vi "TIFF camera test.vi"(8 "Gain":i32 min=0 max=2000 step=1, 9 "Exposure time (ms)":dbl=100.0 min=1.0 max=10000.0 step=1.0) -> (2 "Image out":T1(plugin-control))   [LabVIEW 2017]
uses:
  <vilib>/vision/Image Controls.llb/IMAQ Image.ctl
panel:
  in  "TIF file path":path=path "c:/test.avi"
  in  "stop":bool
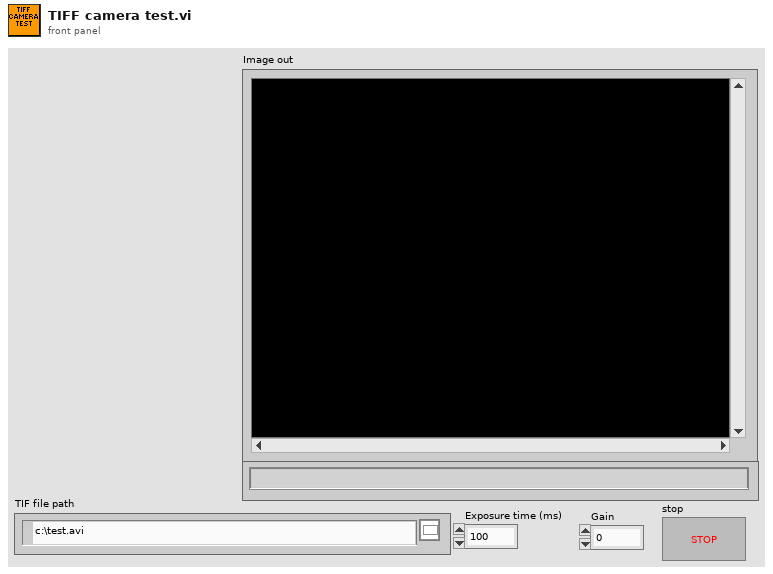
[diagram p1: front panel]
types:
  T1 = typedef "IMAQ Image.ctl" = refnum<image>
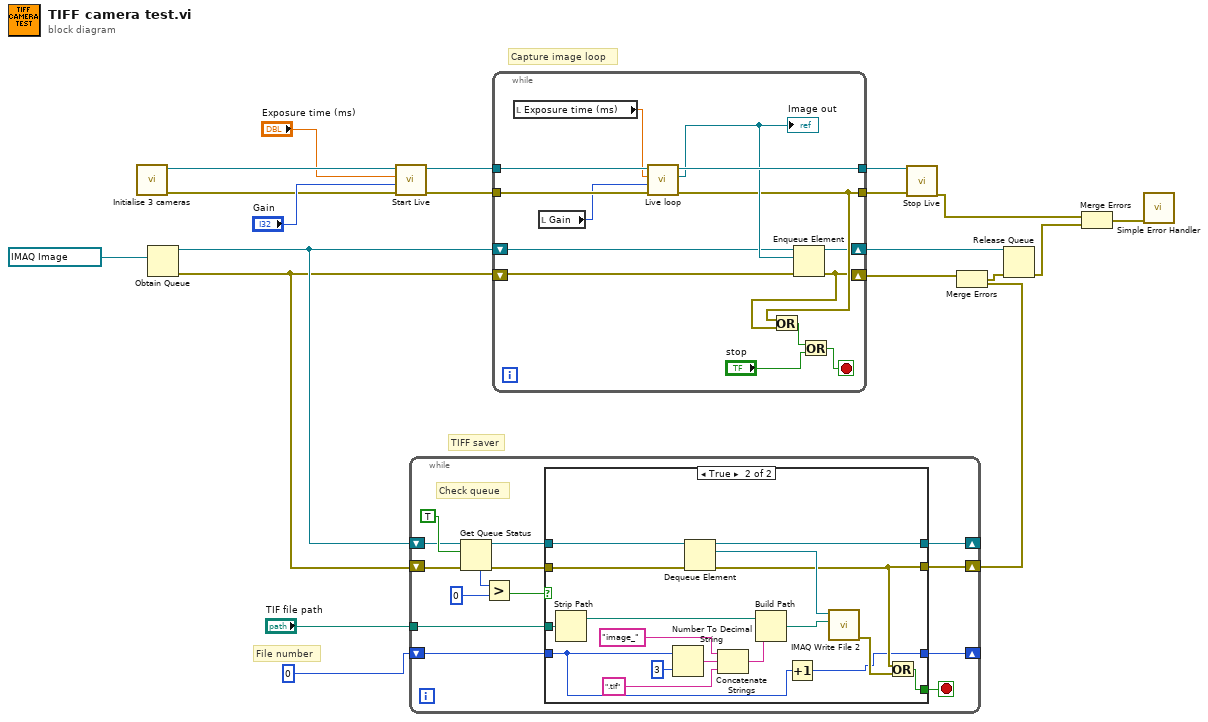
[diagram p0: block diagram]
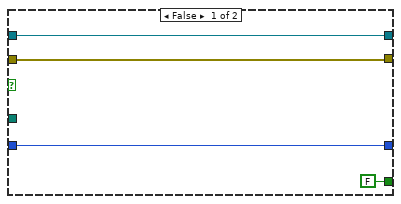
[diagram p2: hidden frame]
diagram:
  # "File number"
  # "TIFF saver"
  # "Capture image loop"
  n1 = call "Initialise 3 cameras.vi"() -> ("Error Out"=w17:errorcluster, "Red camera ref"=w20:refnum<k24>)  [unwired: 8 in, 2 out]
  n2 = Obtain Queue(element data type=T1 refnum ("Image out")) -> (queue out=w5:refnum<queue>, error out=w4:errorcluster)  [unwired: 4 in, 1 out]
  n3 = call "Start Live.vi"("Error In"=w17, "Gain in"="Gain", "Exposure time (ms)"="Exposure time (ms)", "Camera reference in"=w20) -> ("Error Out"=w13:errorcluster, "Camera reference out"=w14:refnum<k24>)  [unwired: 5 in]
  n4 = while {
    shift-right: [w34] -> _
    shift-left: w5 -> [w21]
    shift-right: [w31] -> w3
    shift-left: w4 -> [w24]
    tunnel: "TIF file path" -> [w33]
    shift-right: [w26] -> _
    shift-left: 0 -> [w30]
    stop <- w32 stop-if-true
    # "Check queue"
    n5 = Get Queue Status(queue=w21, return elements? (F)=TRUE, error in (no error)=w24) -> (queue out=w22:refnum<queue>, error out=w23:errorcluster, # elements in queue=w28:i32)  [unwired: 5 out]
    n6 = Greater?(x=w28, y=0) -> (0:w25:bool)
    n7 = case shown="True" w25 {
      tunnel: w22 -> [w38 w55]
      tunnel: w23 -> [w37 w54]
      tunnel: [w38 w53] -> w34
      tunnel: w33 -> [_ w52]
      tunnel: [FALSE w43] -> w32
      tunnel: [w37 w42] -> w31
      tunnel: w30 -> [w36 w40]
      tunnel: [w36 w39] -> w26
      frame False {
      }
      frame True {
        n8 = Strip Path(path=w52) -> (stripped path=w51:path)  [unwired: 1 out]
        n9 = Number To Decimal String(number=w40, width (-)=i16 3) -> (decimal integer string=w49:string)
        n10 = Dequeue Element(queue=w55, error in (no error)=w54) -> (queue out=w53:refnum<queue>, element=w44:T1, error out=w42:errorcluster)  [unwired: 1 in, 1 out]
        n11 = Concatenate Strings("image_", w49, ".tif") -> (w46:string)
        n12 = Build Path(base path=w51, name or relative path=w46) -> (appended path=w45:path)
        n13 = Increment(x=w40) -> (x+1=w39:i32)
        n14 = call-poly "IMAQ Write File 2"("File Path"=w45, "Image"=w44) -> ("error out"=w41:errorcluster)  [unwired: 8 in, 1 out]
        n15 = Or(x=w42, y=w41) -> (x .or. y?=w43:bool)
      }
    }
  }
  n16 = while {
    tunnel: [w58] -> w16
    tunnel: [w69] -> w15
    tunnel: w14 -> [w68]
    tunnel: w13 -> [w67]
    shift-right: [w57] -> w11
    shift-left: w5 -> [w60]
    shift-right: [w56] -> w9
    shift-left: w4 -> [w59]
    stop <- w62 stop-if-true
    n17 = local read "Exposure time (ms)"() -> (w66:dbl)
    n18 = local read "Gain"() -> (w65:i32)
    n19 = call "Live loop.vi"("Error In"=w67, "Gain"=w65, "Exposure time (ms)"=w66, "Camera reference in"=w68) -> ("Error Out"=w58:errorcluster, "Image out"=w61:T1, "Camera reference out"=w69:refnum<k24>)  [unwired: 4 in]
    "Image out" <- w61
    n20 = Enqueue Element(queue=w60, element=w61, error in (no error)=w59) -> (queue out=w57:refnum<queue>, error out=w56:errorcluster)  [unwired: 1 in, 1 out]
    n21 = Or(x=w58, y=w56) -> (x .or. y?=w64:bool)
    n22 = Or(x=w64, y="stop") -> (x .or. y?=w62:bool)
  }
  n23 = call "Stop Live.vi"("Camera reference in"=w15, "Error In"=w16) -> ("Error Out"=w8:errorcluster)  [unwired: 16 in, 1 out]
  n24 = Merge Errors(w9, w3) -> (w10:errorcluster)
  n25 = Release Queue(queue=w11, error in (no error)=w10) -> (error out=w7:errorcluster)  [unwired: 1 in, 2 out]
  n26 = Merge Errors(w8, w7) -> (w6:errorcluster)
  n27 = call <vilib>:"Simple Error Handler.vi"("error in (no error)"=w6) -> ()  [unwired: 4 in, 5 out]
